vi "_pulse2deg.vi"(11 "Pulse":i32[](array[numeric])) -> (3 "Deg":dbl[](array[numeric]))   [LabVIEW 2021, in "System.lvclass"]
uses:
  System.lvclass
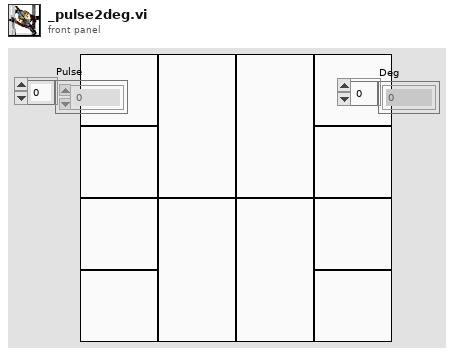
[diagram p1: front panel]
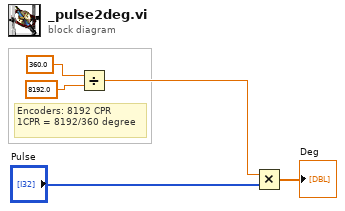
[diagram p0: block diagram]
diagram:
  # "Encoders: 8192 CPR\n1CPR = 8192/360 degree"
  n1 = Divide(x=360.0, y=8192.0) -> (x/y=w3:dbl)
  n2 = Multiply(x=w3, y="Pulse") -> (x*y=→"Deg":dbl[])
